vi "fileformatGlobal.vi"(1 "changed":bool, 2 "Fileformat":enum16{"Herty", "Ken", "SPC130", "HydraHarp"}(ring)) -> (0 "fileformat out":enum16{"Herty", "Ken", "SPC130", "HydraHarp"}(ring))   [LabVIEW 2009]
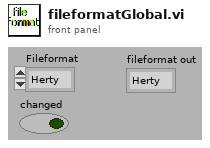
[diagram p1: front panel]
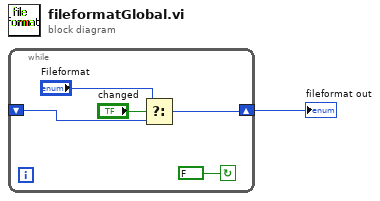
[diagram p0: block diagram]
diagram:
  n1 = while {
    shift-right: [w3] -> w1
    shift-left: _ -> [w4]
    stop <- FALSE continue-if-true
    n2 = Select(t="Fileformat", s="changed", f=w4) -> (s? t:f=w3:enum16{"Herty", "Ken", "SPC130", "HydraHarp"})
  }
  "fileformat out" <- w1
